vi "Find LV Class Ref.vi"(2 "error in (no error)":errorcluster, 3 "Item ID":string, 4 "Expected Project":refnum<vi>) -> (0 "error out":errorcluster, 1 "LVClassLibrary Refnum":refnum<vi>)   [LabVIEW 2020, in "Choose Implementation Dialog.lvlib"]
uses:
  Choose Implementation Dialog.lvlib
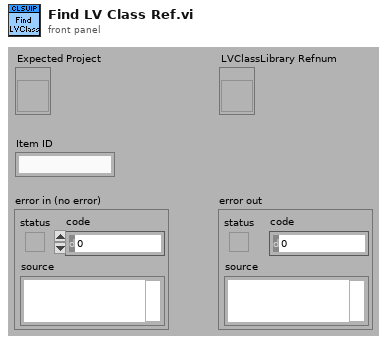
[diagram p1: front panel]
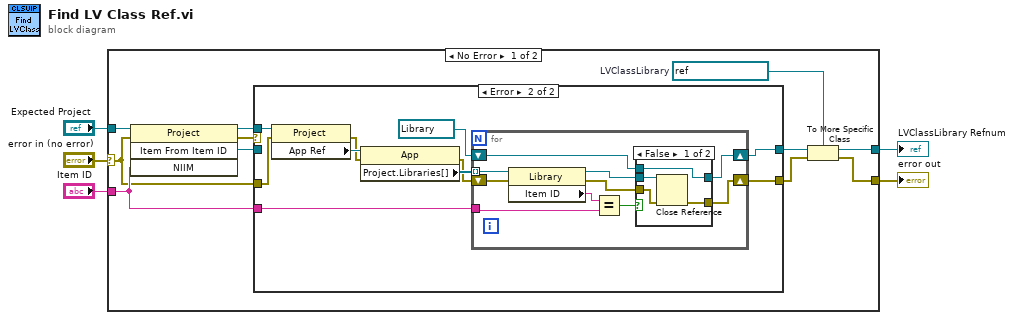
[diagram p0: block diagram]
diagram:
  n1 = case shown="No Error" "error in (no error)" {
    selector: "error in (no error)" -> [w6 w45]
    tunnel: "Expected Project" -> [w16 _]
    tunnel: [w12 w45] -> w1
    tunnel: "Item ID" -> [w8 _]
    tunnel: [w13 _] -> w2
    frame No Error {
      w14 = refnum<vi> refnum  # LVClassLibrary
      n2 = invoke class="Project" method="Item From Item ID"(reference=w16, error in=w6, "NIIM"=w8) -> (reference out=w11:refnum<vi>, error out=w15:errorcluster, "GetItemFromNIIM"=w10:refnum<vi>)  [unwired: 1 in, 1 out]
      n3 = case shown="Error" w15 {
        tunnel: w11 -> [_ w28]
        tunnel: w10 -> [w18 _]
        tunnel: [w18 w25] -> w9
        tunnel: w8 -> [_ w27]
        tunnel: [w17 w20] -> w7
        tunnel: w6 -> [w17 w19]
        frame No Error {
        }
        frame Error {
          n4 = property class="Project"(reference=w28, error in=w19) -> (error out=w21:errorcluster, "App Ref"=w22:refnum<vi>)  [unwired: 1 out]
          n5 = property class="App"(reference=w22, error in=w21) -> (error out=w23:errorcluster, "Project.Libraries[]"=w24:refnum<vi>[])  [unwired: 1 out]
          n6 = for {
            tunnel: w24 -> [w38] mode=indexing
            shift-right: [w31] -> w25
            shift-left: refnum<vi> refnum ("GetItemFromNIIM") -> [w33]
            tunnel: w27 -> [w35]
            shift-right: [w29] -> w20
            shift-left: w23 -> [w37]
            n7 = property class="Library"(reference=w38, error in=w37) -> (reference out=w32:refnum<vi>, error out=w30:errorcluster, "Item ID"=w36:string)
            n8 = Equal?(x=w36, y=w35) -> (x = y?=w34:bool)
            n9 = case shown="False" w34 {
              tunnel: w33 -> [w41 _]
              tunnel: w32 -> [w42 w44]
              tunnel: [w41 w44] -> w31
              tunnel: w30 -> [w40 w43]
              tunnel: [w39 w43] -> w29
              frame False {
                n10 = Close Reference(reference=w42, error in (no error)=w40) -> (error out=w39:errorcluster)
              }
              frame True {
              }
            }
          }
        }
      }
      n11 = To More Specific Class(target class=w14, reference=w9, error in=w7) -> (specific class reference=w13:refnum<vi>, error out=w12:errorcluster)
    }
    frame Error {
    }
  }
  "error out" <- w1
  "LVClassLibrary Refnum" <- w2
